vi "routine1.vi"(9 "amp1":dbl, 10 "section":i16, 11 "theta":dbl) -> (2 "done":i16, 3 "x_d1":dbl)   [LabVIEW 2013]
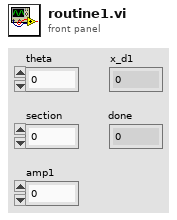
[diagram p1: front panel]
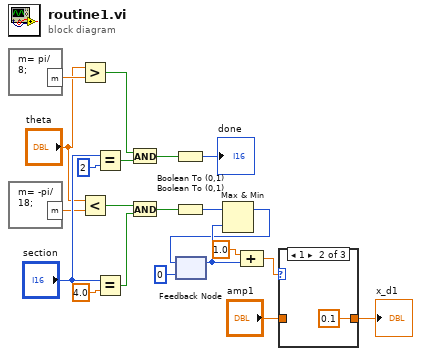
[diagram p0: block diagram]
diagram:
  n1 = formula code="m= pi/8;"() -> ("m"=w13:dbl)
  n2 = formula code="m= -pi/18;"() -> ("m"=w8:dbl)
  n3 = Greater?(x="theta", y=w13) -> (0:w12:bool)
  n4 = Less?(x="theta", y=w8) -> (x < y?=w7:bool)
  n5 = Equal?(x="section", y=i16 2) -> (x = y?=w14:bool)
  n6 = Equal?(x="section", y=4.0) -> (x = y?=w9:bool)
  n7 = And(x=w12, y=w14) -> (x .and. y?=w17:bool)
  n8 = And(x=w7, y=w9) -> (x .and. y?=w6:bool)
  n9 = Boolean To (0,1)(Boolean=w17) -> (0, 1=→"done":i16)
  n10 = Boolean To (0,1)(Boolean=w6) -> (0, 1=w5:i16)
  n11 = feedback #1(i16 0) -> (w4:i16)
  n12 = Max & Min(x=w5, y=w4) -> (max(x,y)=w3:i16)  [unwired: 1 out]
  n13 = feedback-in #1(w3) -> ()
  n14 = Compound Arithmetic op=unknown(1.0 ("value"), w4) -> (w19:dbl)
  n15 = case shown="1" w19 {
    tunnel: [_ 0.1 w23] -> w21
    tunnel: "amp1" -> [_ _ w23]
    frame 0, Default {
    }
    frame 1 {
    }
    frame 2 {
    }
  }
  "x_d1" <- w21
